vi "Project Root.vi"() -> (0 "Project Root":path)   [LabVIEW 2017, in "Scripts.lvlib"]
doc: "Gets the Project Root. The project root, <project root>, is the folder containing the LabVIEW Project file (.lvproj) for this VI."
uses:
  Scripts.lvlib
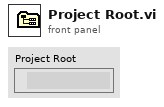
[diagram p1: front panel]
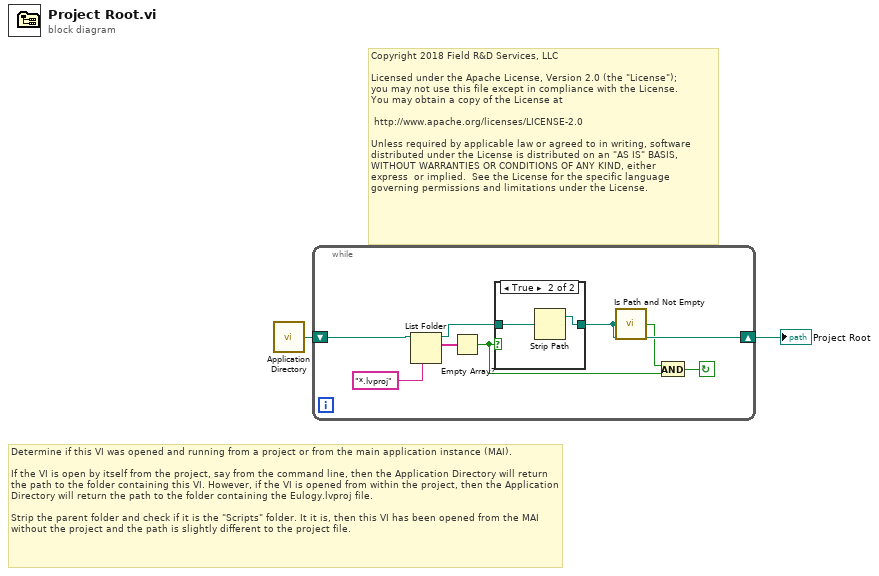
[diagram p0: block diagram]
diagram:
  # "Copyright 2018 Field R&D Services, LLC\n\nLicensed under the Apache License, Version 2.0 (the \"License\");\nyou may not use this file except in compliance with the License.\nYou may obtain a copy of the License at\n\n\thttp://www.apache.org/licenses/LICENSE-2.0\n\nUnless required by applicable law or agreed to in writing, software\ndistributed under the License is distributed on an \"AS IS\" BASIS,\nWITHOUT WARRANTIES OR CONDITIONS OF ANY KIND, either \nexpress  or implied.  See the License for the specific language \ngoverning permissions and limitations under the License."
  # "Determine if this VI was opened and running from a project or from the main application instance (MAI).\n\nIf the VI is open by itself from the project, say from the command line, then the Application Directory will return the path to the folder containing this VI. However, if the VI is opened from within the project, then the Application Directory will return the path to the folder containing the Eulogy.lvproj file. \n\nStrip the parent folder and check if it is the \"Scripts\" folder. It it is, then this VI has been opened from the MAI without the project and the path is slightly different to the project file."
  n1 = call <vilib>:"Application Directory.vi"() -> ("Application Directory"=w2:path)
  n2 = while {
    shift-right: [w6] -> w1
    shift-left: w2 -> [w10]
    stop <- w3 continue-if-true
    n3 = List Folder(path=w10, pattern="*.lvproj") -> (path out=w8:path, filenames=w7:string[])  [unwired: 2 in, 2 out]
    n4 = Empty Array?(array=w7) -> (empty?=w4:bool)
    n5 = case shown="True" w4 {
      tunnel: [w11 w13] -> w6
      tunnel: w8 -> [w11 w12]
      frame False {
      }
      frame True {
        n6 = Strip Path(path=w12) -> (stripped path=w13:path)  [unwired: 1 out]
      }
    }
    n7 = call <vilib>:"Is Path and Not Empty.vi"("path"=w6) -> ("Is Path and Not Empty?"=w5:bool)  [unwired: 4 in]
    n8 = And(x=w5, y=w4) -> (x .and. y?=w3:bool)
  }
  "Project Root" <- w1
